vi "Tosca-Apply Stimulus Condition.vi"(0 "Tosca":refnum<class "Parameters.lvclass">, 1 "SCL":T1[](array[typedef]), 9 "Flag names":string[](array[string]), 11 "error in (no error)":errorcluster, 12 "SCL index":i32) -> (2 "text":string, 3 "StimCon Element":T1, 4 "Tosca out":refnum<class "Parameters.lvclass">, 15 "error out":errorcluster)   [LabVIEW 2020]
uses:
  Typedefs/Tosca-SCL Element.ctl
  Typedefs/Tosca-Schedule Mode.ctl
  Typedefs/Tosca-Event Type.ctl
  Classes/Parameters/Parameters.lvclass
  Classes/Parameters/Parameters.lvclass/Parameters.ctl
  Classes/Parameters/Read Input Events.vi
  Classes/Parameters/Read Pretrial.vi
  Classes/Parameters/Read Flowchart.vi
  Classes/Parameters/Read DAQ.vi
  Classes/Parameters/Write Pretrial.vi
  Classes/Parameters/Write Flowchart.vi
  Sub VIs/Tosca-Globals.vi
  Classes/State/State.lvclass
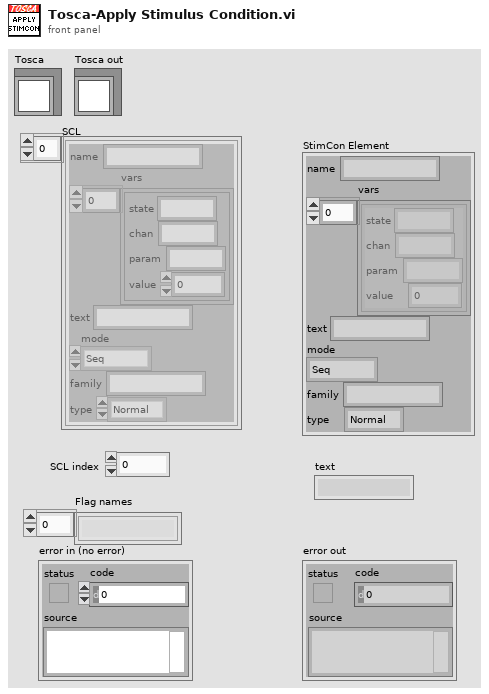
[diagram p1: front panel]
types:
  T1 = typedef "Tosca-SCL Element.ctl" = cluster{"name":string, "vars":cluster{"state":string, "chan":string, "param":string, "value":dbl}[], "text":string, "mode":T2, "family":string, "type":T3}
  T2 = typedef "Tosca-Schedule Mode.ctl" = enum16{"Seq", "CS+/CS-", "Adapt"}
  T3 = typedef "Tosca-Event Type.ctl" = enum16{"Normal", "CS+", "CS-"}
  T4 = typedef "Tosca-Pretrial Spec.ctl" = cluster{"Path":path, "Args":string[]}
  T5 = typedef "Parameters.lvclass/DAQ.ctl" = cluster{"AO Fs (Hz)":dbl, "DO Fs (Hz)":dbl, "Poll Rate (Hz)":dbl, "Baseline (s)":dbl}
  T6 = cluster{"state":string, "chan":string, "param":string, "value":dbl}[]
  T7 = typedef "Tosca-Input Event.ctl" = cluster{"Name":string, "Criteria":T8[], "Operators":enum16{"AND", "OR"}[], "Accumulator":T10}
  T8 = typedef "Tosca-Input Criterion.ctl" = cluster{"DigInput":i32, "State":T9, "Time (ms)":i32, "Name":string}
  T9 = typedef "Logic State.ctl" = enum16{"Low", "High", "Rising", "Falling"}
  T10 = typedef "Tosca-Accumulator.ctl" = cluster{"active":bool, "N":i32, "T":dbl, "Imax":dbl, "latency":dbl}
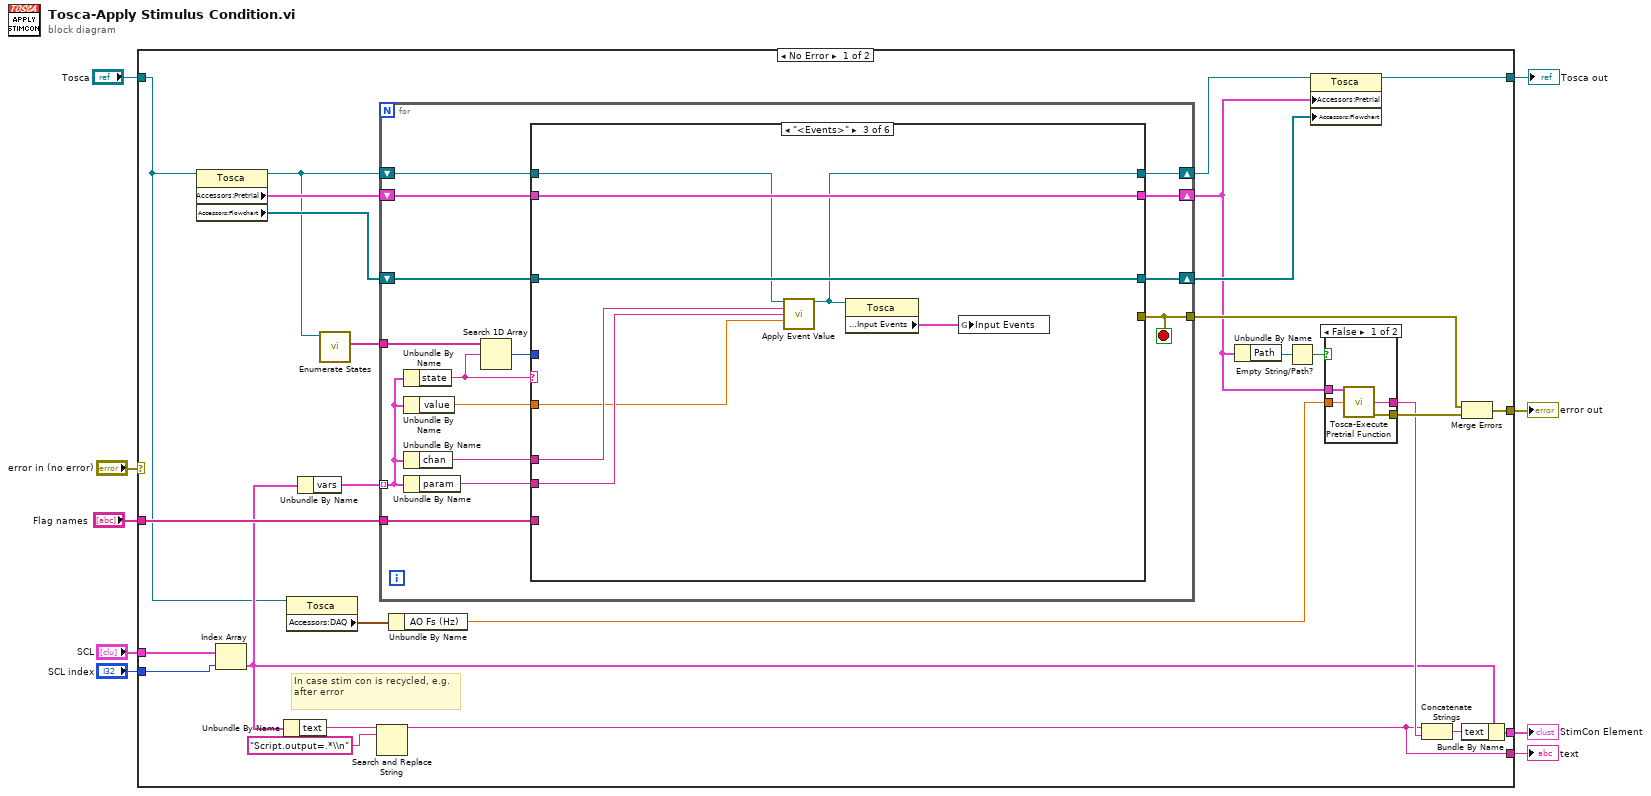
[diagram p0: block diagram]
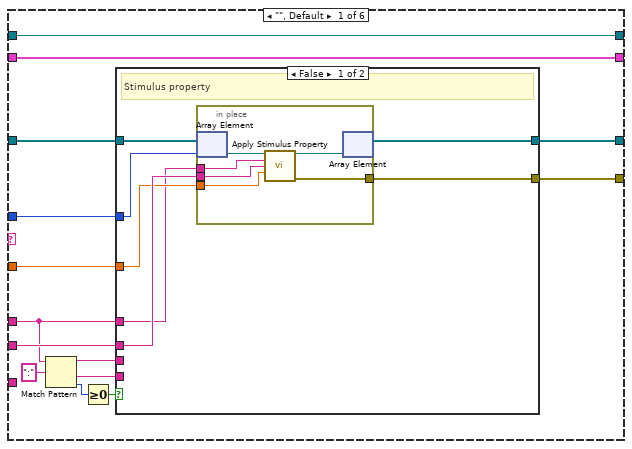
[diagram p2: hidden frame]
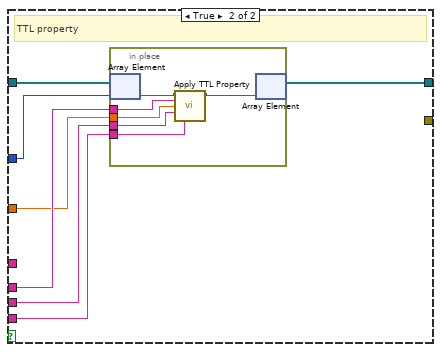
[diagram p3: hidden frame]
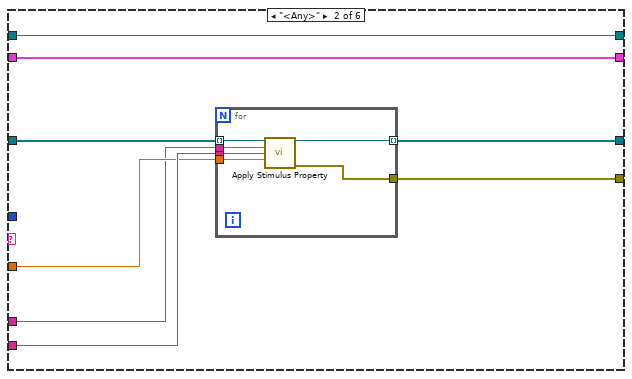
[diagram p4: hidden frame]
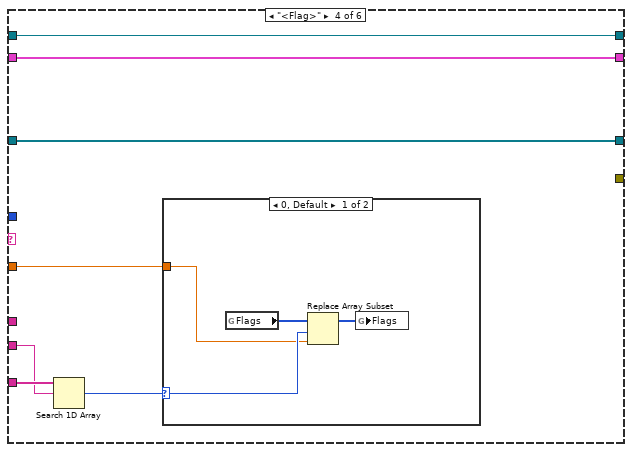
[diagram p5: hidden frame]
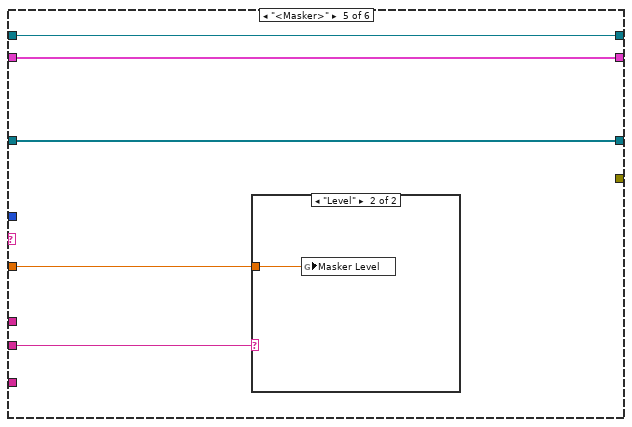
[diagram p7: hidden frame]
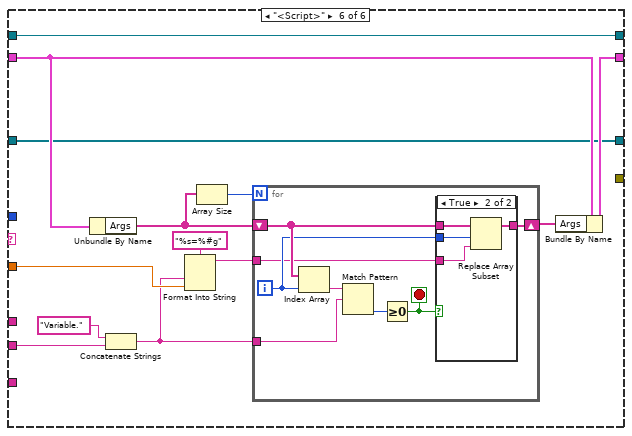
[diagram p9: hidden frame]
diagram:
  n1 = case shown="No Error" "error in (no error)" {
    selector: "error in (no error)" -> [_ w162]
    tunnel: [w15 w162] -> w8
    tunnel: "SCL" -> [w36 _]
    tunnel: [w34 _] -> w6
    tunnel: "SCL index" -> [w35 _]
    tunnel: [w23 _] -> w4
    tunnel: "Flag names" -> [w24 _]
    tunnel: "Tosca" -> [w17 w161]
    tunnel: [w16 w161] -> w1
    frame No Error {
      # "In case stim con is recycled, e.g. after error"
      n2 = property class="Tosca"(reference=w17) -> (reference out=w11:refnum<class "Parameters.lvclass">, "Accessors:Pretrial"=w20:T4, "Accessors:Flowchart"=w18:refnum<class "State.lvclass">[])  [unwired: 1 in, 1 out]
      n3 = Index Array(array=w36, index=w35) -> (element=w22:T1)
      n4 = Unbundle By Name(w22) -> ("text"=w26:string)
      n5 = property class="Tosca"(reference=w17) -> ("Accessors:DAQ"=w21:T5)  [unwired: 1 in, 2 out]
      n6 = Unbundle By Name(w22) -> ("vars"=w33:T6)
      n7 = call "Enumerate States.vi"("Tosca in"=w11) -> ("Names"=w19:string[])  [unwired: 8 in, 2 out]
      n8 = Search and Replace String(input string=w26, search string="Script.output=.*\\n") -> (result string=w23:string)  [unwired: 6 in, 3 out]
      n9 = for {
        tunnel: w33 -> [w48] mode=indexing
        tunnel: w19 -> [w51]
        shift-right: [w43] -> w12
        shift-left: w20 -> [w44]
        tunnel: w24 -> [w42]
        shift-right: [w40] -> w13
        shift-left: w18 -> [w41]
        tunnel: [w39] -> w14
        shift-right: [w37] -> w10
        shift-left: w11 -> [w38]
        stop <- w39 stop-if-true
        n10 = Unbundle By Name(w48) -> ("state"=w45:string)
        n11 = Unbundle By Name(w48) -> ("value"=w47:dbl)
        n12 = Unbundle By Name(w48) -> ("chan"=w46:string)
        n13 = Unbundle By Name(w48) -> ("param"=w49:string)
        n14 = Search 1D Array(1D array=w51, element=w45) -> (index of element=w50:i32)  [unwired: 1 in]
        n15 = case shown="\"<Events>\"" w45 {
          tunnel: w50 -> [w61 _ _ _ _ _]
          tunnel: w49 -> [w60 w99 w109 w118 w129 w143]
          tunnel: w47 -> [w59 w98 w108 w116 w128 w140]
          tunnel: w46 -> [w56 w96 w110 _ _ _]
          tunnel: w44 -> [w57 w97 w113 w120 w127 w139]
          tunnel: [w57 w97 w113 w120 w127 w137] -> w43
          tunnel: w42 -> [_ _ _ w119 _ _]
          tunnel: w41 -> [w55 w94 w112 w115 w126 w132]
          tunnel: [w54 w93 w112 w115 w126 w132] -> w40
          tunnel: [w53 w95 _ _ _ _] -> w39
          tunnel: w38 -> [w52 w92 w111 w114 w125 w131]
          tunnel: [w52 w92 w107 w114 w125 w131] -> w37
          frame "", Default {
            n16 = Match Pattern(string=w56, regular expression=":") -> (before substring=w58:string, after substring=w62:string, offset past match=w64:i32)  [unwired: 1 in, 1 out]
            n17 = Greater Or Equal To 0?(x=w64) -> (x >= 0?=w63:bool)
            n18 = case shown="False" w63 {
              tunnel: w62 -> [_ w82]
              tunnel: w61 -> [w67 w79]
              tunnel: w60 -> [w70 w85]
              tunnel: w59 -> [w69 w84]
              tunnel: w58 -> [_ w83]
              tunnel: w56 -> [w68 _]
              tunnel: w55 -> [w72 w81]
              tunnel: [w71 w80] -> w54
              tunnel: [w66 _] -> w53
              frame False {
                # "Stimulus property"
                n19 = in-place {
                  in-place-border: w70 -> [w74]
                  in-place-border: w69 -> [w76]
                  in-place-border: w68 -> [w75]
                  in-place-border: [w73] -> w66
                  n20 = in-place-array #1(w72, w67) -> (w78:refnum<class "State.lvclass">)
                  n21 = call "Apply Stimulus Property.vi"("State in"=w78, "chan"=w75, "param"=w74, "value"=w76) -> ("State out"=w77:refnum<class "State.lvclass">, "error out"=w73:errorcluster)  [unwired: 10 in]
                  n22 = in-place-array #1(w77) -> (w71:refnum<class "State.lvclass">[])  [unwired: 1 out]
                }
              }
              frame True {
                # "TTL property"
                n23 = in-place {
                  in-place-border: w85 -> [w89]
                  in-place-border: w84 -> [w88]
                  in-place-border: w83 -> [w87]
                  in-place-border: w82 -> [w86]
                  n24 = in-place-array #2(w81, w79) -> (w91:refnum<class "State.lvclass">)
                  n25 = call "Apply TTL Property.vi"("State in"=w91, "param"=w89, "value"=w88, "chan"=w87, "TTL name"=w86) -> ("State out"=w90:refnum<class "State.lvclass">)  [unwired: 9 in, 1 out]
                  n26 = in-place-array #2(w90) -> (w80:refnum<class "State.lvclass">[])  [unwired: 1 out]
                }
              }
            }
          }
          frame "<Any>" {
            n27 = for {
              tunnel: w99 -> [w105]
              tunnel: w98 -> [w104]
              tunnel: w96 -> [w103]
              tunnel: [w102] -> w95
              tunnel: w94 -> [w101] mode=indexing
              tunnel: [w100] -> w93 mode=indexing
              n28 = call "Apply Stimulus Property.vi"("State in"=w101, "chan"=w103, "param"=w105, "value"=w104) -> ("State out"=w100:refnum<class "State.lvclass">, "error out"=w102:errorcluster)  [unwired: 10 in]
            }
          }
          frame "<Events>" {
            n29 = call "Apply Event Value.vi"("Tosca in"=w111, "Event"=w110, "Criterion"=w109, "Value"=w108) -> ("Tosca out"=w107:refnum<class "Parameters.lvclass">)  [unwired: 10 in, 1 out]
            n30 = property class="Tosca"(reference=w107) -> ("Accessors:Input Events"=w106:T7[])  [unwired: 1 in, 2 out]
            n31 = global write "Tosca-Globals.vi" "Input Events"(w106) -> ()
          }
          frame "<Flag>" {
            n32 = Search 1D Array(1D array=w119, element=w118) -> (index of element=w117:i32)  [unwired: 1 in]
            n33 = case shown="0, Default" w117 {
              selector: w117 -> [w123 _]
              tunnel: w116 -> [w122 _]
              frame 0, Default {
                n34 = global read "Tosca-Globals.vi" "Flags"() -> (w124:i32[])
                n35 = Replace Array Subset(array=w124, new element=w122, index=w123) -> (w121:i32[])
                n36 = global write "Tosca-Globals.vi" "Flags"(w121) -> ()
              }
              frame -1 {
              }
            }
          }
          frame "<Masker>" {
            n37 = case shown="\"Level\"" w129 {
              tunnel: w128 -> [_ w130]
              frame "", Default {
              }
              frame "Level" {
                n38 = global write "Tosca-Globals.vi" "Masker Level"(w130) -> ()
              }
            }
          }
          frame "<Script>" {
            n39 = Unbundle By Name(w139) -> ("Args"=w134:string[])
            n40 = Concatenate Strings("Variable.", w143) -> (w138:string)
            n41 = Format Into String(format string="%s=%#g", w138, w140) -> (resulting string=w133:string)  [unwired: 2 in, 1 out]
            n42 = Array Size(array=w134) -> (size(s)=w135:i32)
            n43 = for {
              N: w135 -> [_]
              shift-right: [w148] -> w136
              shift-left: w134 -> [w149]
              tunnel: w138 -> [w145]
              tunnel: w133 -> [w144]
              i -> [w146]
              stop <- w147 stop-if-true
              n44 = Index Array(array=w149, index=w146) -> (element=w151:string)
              n45 = Match Pattern(string=w151, regular expression=w145) -> (offset past match=w150:i32)  [unwired: 1 in, 3 out]
              n46 = Greater Or Equal To 0?(x=w150) -> (x >= 0?=w147:bool)
              n47 = case shown="True" w147 {
                tunnel: w149 -> [w152 w156]
                tunnel: [w152 w155] -> w148
                tunnel: w146 -> [_ w154]
                tunnel: w144 -> [_ w153]
                frame False {
                }
                frame True {
                  n48 = Replace Array Subset(array=w156, new element=w153, index=w154) -> (w155:string[])
                }
              }
            }
            n49 = Bundle By Name(cluster=w139, "Args"=w136) -> (w137:T4)
          }
        }
      }
      n50 = Unbundle By Name(w21) -> ("AO Fs (Hz)"=w29:dbl)
      n51 = Unbundle By Name(w12) -> ("Path"=w31:path)
      n52 = Empty String/Path?(string/path=w31) -> (empty?=w32:bool)
      n53 = property class="Tosca"(reference=w10, "Accessors:Pretrial"=w12, "Accessors:Flowchart"=w13) -> (reference out=w16:refnum<class "Parameters.lvclass">)  [unwired: 1 in, 1 out]
      n54 = case shown="False" w32 {
        tunnel: [w160 _] -> w30
        tunnel: w12 -> [w159 _]
        tunnel: w29 -> [w158 _]
        tunnel: [w157 _] -> w27
        frame False {
          n55 = call "Tosca-Execute Pretrial Function.vi"("Pretrial in"=w159, "Fs"=w158) -> ("output"=w157:string, "error out"=w160:errorcluster)  [unwired: 12 in]
        }
        frame True {
        }
      }
      n56 = Concatenate Strings(w23, w27) -> (w28:string)
      n57 = Merge Errors(w14, w30) -> (w15:errorcluster)
      n58 = Bundle By Name(cluster=w22, "text"=w28) -> (w34:T1)
    }
    frame Error {
    }
  }
  "error out" <- w8
  "StimCon Element" <- w6
  "text" <- w4
  "Tosca out" <- w1
